vi "DriveSpeedOutput.vi"   [LabVIEW 2019]
uses:
  refnums.vi
  81ed1d8f-b977-4dba-a2ed-962307b4cc63.vi
  outputs.vi
  dsdata.vi
  sensors.vi
  GRNF_GenericMotor.vi
types:
  T1 = typedef "WPI_MotorControlDeviceRef.ctl" = cluster{"DeviceStatus":errorcluster, "Type":T2, "PWM":cluster{"PWM Channel":T3, "DeadBand":T4}, "CAN":cluster{"Device Number":u8, "SetOutput VI Ref":variant, "GetOutput VI Ref":variant, "Enable VI Ref":variant, "Disable VI Ref":variant, "Data":variant}, "Invert":bool, "DIO PWM":cluster{"PWM \"Enable\" Channel":T3, "DIOChannel":T5, "PWM Rate":dbl}}
  T2 = typedef "WPI_MotorControlType.ctl" = enum16{"PWM", "CAN", "DIO PWM"}
  T3 = typedef "FPGA_DIOPWMChannel.ctl" = enum8{"PWM 0", "PWM 1", "PWM 2", "PWM 3", "PWM 4", "PWM 5", "PWM 6", "PWM 7", "PWM 8", "PWM 9", "PWM MXP 0", "PWM MXP 1", "PWM MXP 2", "PWM MXP 3", "PWM MXP 4", "PWM MXP 5", "PWM MXP 6", "PWM MXP 7", "PWM MXP 8", "PWM MXP 9", "Invalid"}
  T4 = typedef "WPI_PWMDeadband.ctl" = cluster{"Name":string, "maxPositivePwm":i32, "minPositivePwm":i32, "centerPwm":i32, "maxNegativePwm":i32, "minNegativePwm":i32, "angularRange":u16}
  T5 = typedef "FPGA_DIOChannel.ctl" = enum8{"DIO 0", "DIO 1", "DIO 2", "DIO 3", "DIO 4", "DIO 5", "DIO 6", "DIO 7", "DIO 8", "DIO 9", "DIO MXP 0", "DIO MXP 1", "DIO MXP 2", "DIO MXP 3", "DIO MXP 4", "DIO MXP 5", "DIO MXP 6", "DIO MXP 7", "DIO MXP 8", "DIO MXP 9", "DIO MXP 10", "DIO MXP 11", "DIO MXP 12", "DIO MXP 13", "DIO MXP 14", "DIO MXP 15", "SPI Port CS1", "SPI Port CS2", "SPI Port CS3", "SPI Port MISO", "SPI Port MOSI", "Invalid"}
  T6 = typedef "WPI_DriverStationRobotMode2.ctl" = enum16{"Autonomous Disabled", "Autonomous Enabled", "Teleop Disabled", "Teleop Enabled", "Disconnected", "Finish", "Test Disabled", "Test Enabled", "Emergency Stopped"}
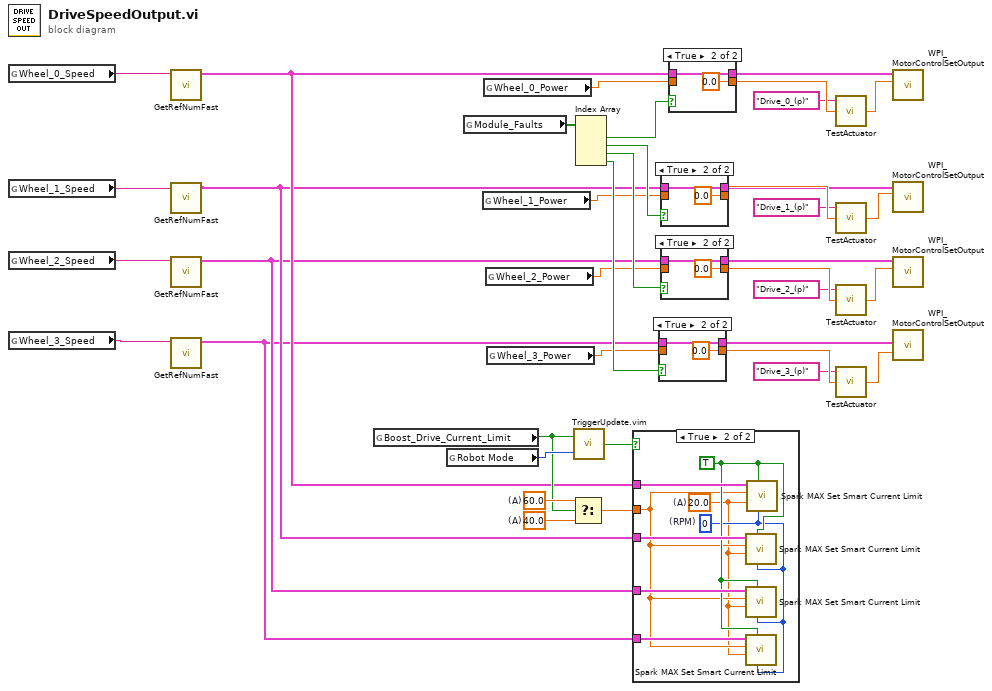
[diagram p0: block diagram]
diagram:
  w13 = 40.0  # (A)
  w12 = 60.0  # (A)
  n1 = global read "refnums.vi" "Wheel_0_Speed"() -> (w4:string)
  n2 = global read "refnums.vi" "Wheel_1_Speed"() -> (w3:string)
  n3 = global read "refnums.vi" "Wheel_2_Speed"() -> (w2:string)
  n4 = global read "refnums.vi" "Wheel_3_Speed"() -> (w1:string)
  n5 = call-poly "GetRefNumFast.vi"("RefNum Name"=w4) -> ("Device Reference"=w8:T1)  [unwired: 5 in, 1 out]
  n6 = call-poly "GetRefNumFast.vi"("RefNum Name"=w3) -> ("Device Reference"=w7:T1)  [unwired: 5 in, 1 out]
  n7 = call-poly "GetRefNumFast.vi"("RefNum Name"=w2) -> ("Device Reference"=w6:T1)  [unwired: 5 in, 1 out]
  n8 = call-poly "GetRefNumFast.vi"("RefNum Name"=w1) -> ("Device Reference"=w5:T1)  [unwired: 5 in, 1 out]
  n9 = global read "outputs.vi" "Boost_Drive_Current_Limit"() -> (w10:bool)
  n10 = global read "dsdata.vi" "Robot Mode"() -> (w14:T6)
  n11 = global read "sensors.vi" "Module_Faults"() -> (w15:bool[])
  n12 = global read "outputs.vi" "Wheel_1_Power"() -> (w20:dbl)
  n13 = global read "outputs.vi" "Wheel_0_Power"() -> (w18:dbl)
  n14 = global read "outputs.vi" "Wheel_2_Power"() -> (w23:dbl)
  n15 = global read "outputs.vi" "Wheel_3_Power"() -> (w26:dbl)
  n16 = Select(t=w12, s=w10, f=w13) -> (s? t:f=w11:dbl)
  n17 = call "TriggerUpdate.vim"("Robot Mode"=w14, "Trigger"=w10) -> ("Update"=w9:bool)
  n18 = Index Array(array=w15) -> (element #1=w16:bool, element #2=w21:bool, element #3=w24:bool, element #4=w27:bool)  [unwired: 4 in]
  n19 = case shown="True" w9 {
    tunnel: w5 -> [_ w47]
    tunnel: w6 -> [_ w46]
    tunnel: w7 -> [_ w45]
    tunnel: w8 -> [_ w44]
    tunnel: w11 -> [_ w41]
    frame False {
    }
    frame True {
      w40 = 20.0  # (A)
      w42 = u32 0  # (RPM)
      w43 = TRUE ("Linearized Limit Enabled (F)")
      n20 = call <vilib>:"Spark MAX Set Smart Current Limit.vi"("Linear Limit RPM (0)"=w42, "Linearized Limit Enabled (F)"=w43, "Free Speed Current Limit (20A)"=w40, "Primay Current Limit (80A)"=w41, "MotorControlDeviceRef in"=w45) -> ()  [unwired: 5 in, 2 out]
      n21 = call <vilib>:"Spark MAX Set Smart Current Limit.vi"("Linear Limit RPM (0)"=w42, "Linearized Limit Enabled (F)"=w43, "Free Speed Current Limit (20A)"=w40, "Primay Current Limit (80A)"=w41, "MotorControlDeviceRef in"=w46) -> ()  [unwired: 5 in, 2 out]
      n22 = call <vilib>:"Spark MAX Set Smart Current Limit.vi"("Linear Limit RPM (0)"=w42, "Linearized Limit Enabled (F)"=w43, "Free Speed Current Limit (20A)"=w40, "Primay Current Limit (80A)"=w41, "MotorControlDeviceRef in"=w47) -> ()  [unwired: 5 in, 2 out]
      n23 = call <vilib>:"Spark MAX Set Smart Current Limit.vi"("Linear Limit RPM (0)"=w42, "Linearized Limit Enabled (F)"=w43, "Free Speed Current Limit (20A)"=w40, "Primay Current Limit (80A)"=w41, "MotorControlDeviceRef in"=w44) -> ()  [unwired: 5 in, 2 out]
    }
  }
  n24 = case shown="True" w27 {
    tunnel: [w49 w51] -> w25
    tunnel: w5 -> [w49 w51]
    tunnel: [w48 0.0 ("Command")] -> w38
    tunnel: w26 -> [w48 _]
    frame False {
    }
    frame True {
    }
  }
  n25 = case shown="True" w21 {
    tunnel: [w53 w55] -> w19
    tunnel: w7 -> [w53 w55]
    tunnel: [w52 0.0 ("Command")] -> w29
    tunnel: w20 -> [w52 _]
    frame False {
    }
    frame True {
    }
  }
  n26 = case shown="True" w24 {
    tunnel: [w57 w59] -> w22
    tunnel: w6 -> [w57 w59]
    tunnel: [w56 0.0 ("Command")] -> w35
    tunnel: w23 -> [w56 _]
    frame False {
    }
    frame True {
    }
  }
  n27 = case shown="True" w16 {
    tunnel: [w61 w63] -> w17
    tunnel: w8 -> [w61 w63]
    tunnel: [w60 0.0 ("Command")] -> w32
    tunnel: w18 -> [w60 _]
    frame False {
    }
    frame True {
    }
  }
  n28 = call "TestActuator.vi"("Input_Value_Double"=w32, "Actuator_Name"="Drive_0_(p)") -> ("Output_Value_Double"=w33:dbl)  [unwired: 1 in, 2 out]
  n29 = call "TestActuator.vi"("Input_Value_Double"=w29, "Actuator_Name"="Drive_1_(p)") -> ("Output_Value_Double"=w30:dbl)  [unwired: 1 in, 2 out]
  n30 = call "TestActuator.vi"("Input_Value_Double"=w35, "Actuator_Name"="Drive_2_(p)") -> ("Output_Value_Double"=w36:dbl)  [unwired: 1 in, 2 out]
  n31 = call "TestActuator.vi"("Input_Value_Double"=w38, "Actuator_Name"="Drive_3_(p)") -> ("Output_Value_Double"=w39:dbl)  [unwired: 1 in, 2 out]
  n32 = call <vilib>:"WPI_MotorControlSetOutput.vi"("Output"=w33, "MotorControlDevRef"=w17) -> ()  [unwired: 7 in, 3 out]
  n33 = call <vilib>:"WPI_MotorControlSetOutput.vi"("Output"=w30, "MotorControlDevRef"=w19) -> ()  [unwired: 7 in, 3 out]
  n34 = call <vilib>:"WPI_MotorControlSetOutput.vi"("Output"=w36, "MotorControlDevRef"=w22) -> ()  [unwired: 7 in, 3 out]
  n35 = call <vilib>:"WPI_MotorControlSetOutput.vi"("Output"=w39, "MotorControlDevRef"=w25) -> ()  [unwired: 7 in, 3 out]
